vi "Read measurement.vi"(6 "error in":errorcluster, 9 "VISA resource name":refnum<visa-resource-name>) -> (0 "error out":errorcluster, 1 "number":dbl, 2 "Read data":string, 3 "VISA resource name out":refnum<visa-resource-name>)   [LabVIEW 2023, in "Aim TTi 1908P DMM.lvlib"]
uses:
  Aim TTi 1908P DMM.lvlib
  19e38209-455c-425b-9d7c-0b824d84d338.vi
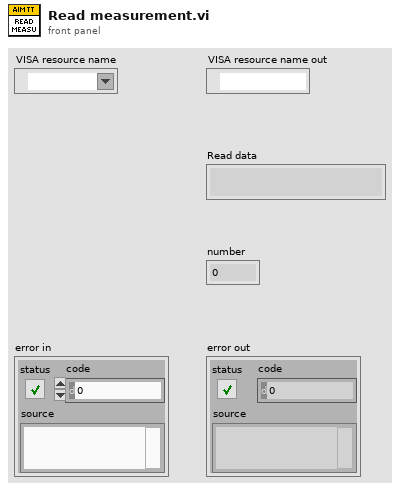
[diagram p1: front panel]
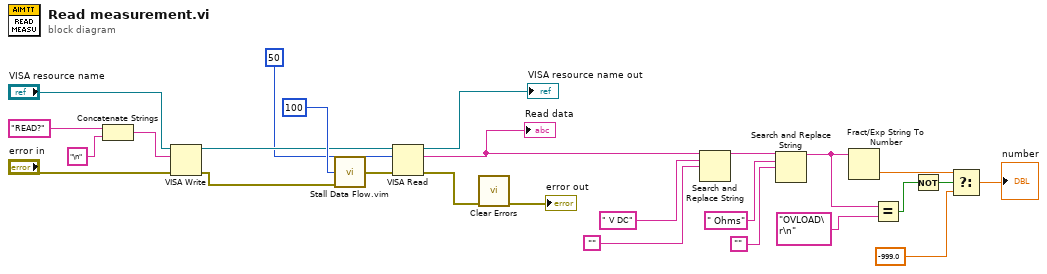
[diagram p0: block diagram]
diagram:
  n1 = Concatenate Strings("READ?" ("Read command"), "\n" ("string")) -> (w21:string)
  n2 = VISA Write(VISA resource name="VISA resource name", write buffer=w21, error in (no error)="error in") -> (VISA resource name out=w3:refnum<visa-resource-name>, error out=w2:errorcluster)  [unwired: 1 out]
  n3 = call "Stall Data Flow.vim"("value in"=w2, "milliseconds to wait"=u32 100) -> ("value out"=w26:errorcluster)  [unwired: 1 out]
  n4 = VISA Read(VISA resource name=w3, byte count=u32 50, error in (no error)=w26) -> (VISA resource name out=→"VISA resource name out":refnum<visa-resource-name>, read buffer=w14:string, error out=w18:errorcluster)  [unwired: 1 out]
  "Read data" <- w14
  n5 = call <vilib>:"Clear Errors.vi"("error in (no error)"=w18) -> ("error out"=→"error out":errorcluster)  [unwired: 5 in, 1 out]
  n6 = Search and Replace String(input string=w14, search string=" V DC", replace string="") -> (result string=w13:string)  [unwired: 5 in, 3 out]
  n7 = Search and Replace String(input string=w13, search string=" Ohms", replace string="") -> (result string=w10:string)  [unwired: 5 in, 3 out]
  n8 = Fract/Exp String To Number(string=w10) -> (number=w8:dbl)  [unwired: 3 in, 1 out]
  n9 = Equal?(x=w10, y="OVLOAD\r\n" ("Read data")) -> (x = y?=w7:bool)
  n10 = Not(x=w7) -> (.not. x?=w4:bool)
  n11 = Select(t=w8, s=w4, f=-999.0) -> (s? t:f=→"number":dbl)
